vi "Remove Routing Channel.vi"(8 "error in (no error)":errorcluster, 10 "Channel Name":string, 11 "Routes Ref in":T1 format="%.0x") -> (0 "error out":errorcluster, 3 "Routes Ref out":T1 format="%.0x")   [LabVIEW 2017, in "SLSC Switch Scripting.lvlib"]
uses:
  SLSC Switch Scripting.lvlib
  <vilib>/NI Veristand/Custom Device API/Custom Device Item Ref.ctl
  <vilib>/NI VeriStand/Custom Device API/Custom Device API.lvlib
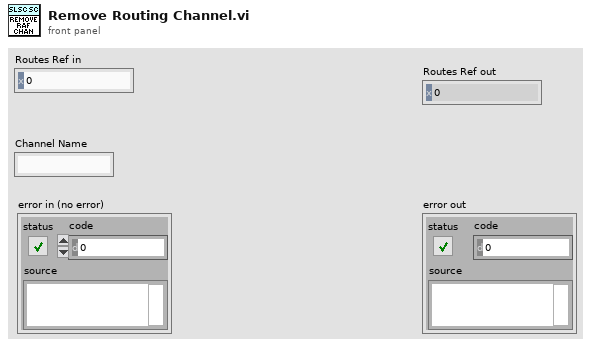
[diagram p1: front panel]
types:
  T1 = typedef "Custom Device API.lvlib/Custom Device Item Ref.ctl" = u64
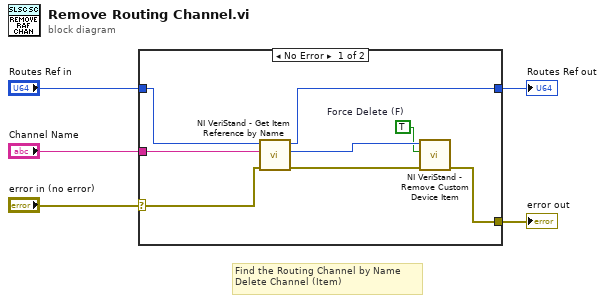
[diagram p0: block diagram]
diagram:
  # "Find the Routing Channel by Name\nDelete Channel (Item)"
  n1 = case shown="No Error" "error in (no error)" {
    selector: "error in (no error)" -> [w12 w15]
    tunnel: [w6 w15] -> w5
    tunnel: [w9 w14] -> w4
    tunnel: "Routes Ref in" -> [w13 w14]
    tunnel: "Channel Name" -> [w11 _]
    frame No Error {
      w7 = TRUE  # Force Delete (F)
      n2 = call <vilib>:"NI VeriStand - Get Item Reference by Name.vi"("error in (no error)"=w12, "Item Name"=w11, "Parent Ref in"=w13) -> ("error out"=w8:errorcluster, "Item Ref"=w10:T1, "Parent Ref out"=w9:T1)  [unwired: 5 in, 1 out]
      n3 = call <vilib>:"NI VeriStand - Remove Custom Device Item.vi"("error in (no error)"=w8, "Force Delete (F)"=w7, "Item Ref in"=w10) -> ("error out"=w6:errorcluster)  [unwired: 7 in, 1 out]
    }
    frame Error {
    }
  }
  "error out" <- w5
  "Routes Ref out" <- w4
